vi "Get Type.vi"(11 "Boolean 1D in":refnum<class "Boolean 1D.lvclass">) -> (3 "Type":string)   [LabVIEW 2020, in "Boolean 1D.lvclass"]
uses:
  <vilib>/gpm_packages/@cs/data-type-serializer/source/Boolean 1D/Boolean 1D.lvclass
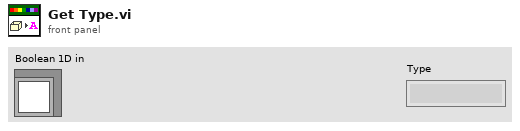
[diagram p1: front panel]
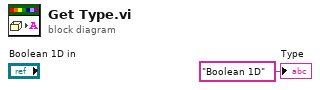
[diagram p0: block diagram]
diagram:
  "Type" <- "Boolean 1D" ("Type")
